vi "ProcessRepository.vi"(0 "reference in":refnum<class "Battery.lvclass">, 1 "Action(ReadRepository)":T1(ring), 5 "Error In":errorcluster) -> (7 "QueueFromProcess":refnum<queue>, 9 "ProcessViRef":refnum<vi>, 11 "ProcessSyncQueue":refnum<queue>, 13 "EventFromProcess":refnum<user-event>, 14 "reference out":refnum<class "Battery.lvclass">, 15 "EventsToProcess":refnum<user-event>, 17 "ProcessAlreadyStarted":bool, 19 "Error Out":errorcluster)   [LabVIEW 2023, in "Battery.lvclass"]
uses:
  Battery.lvclass
  Battery.lvclass/Battery.ctl
  Process.ctl
  Process.vi
panel:
  # "Use this indicator for sending messages to the Process VI"
  # "These indicators are used by the process VIs"
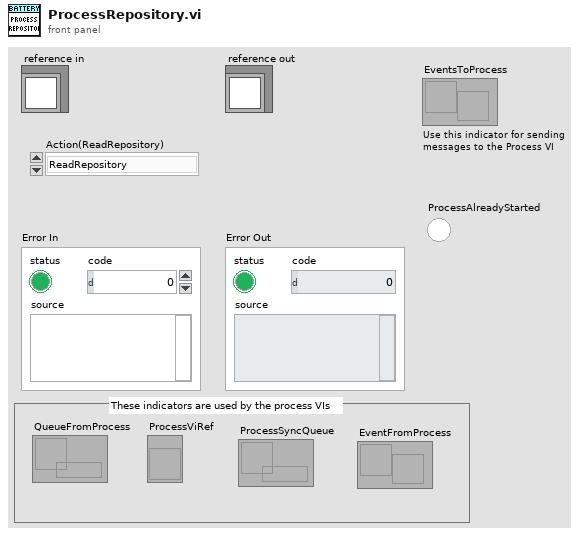
[diagram p1: front panel]
types:
  T1 = enum16{"ReadRepository", "CreateNew", "CreateOrLookUpExisting", "ReadRepositoryAndDestroy"}
  T2 = typedef "Battery.lvclass/Process.ctl" = cluster{"EventsToProcess":refnum<user-event>, "EventFromProcess":refnum<user-event>, "ProcessSyncQueue":refnum<queue>, "ProcessViRef":refnum<vi>, "QueueFromProcess":refnum<queue>}
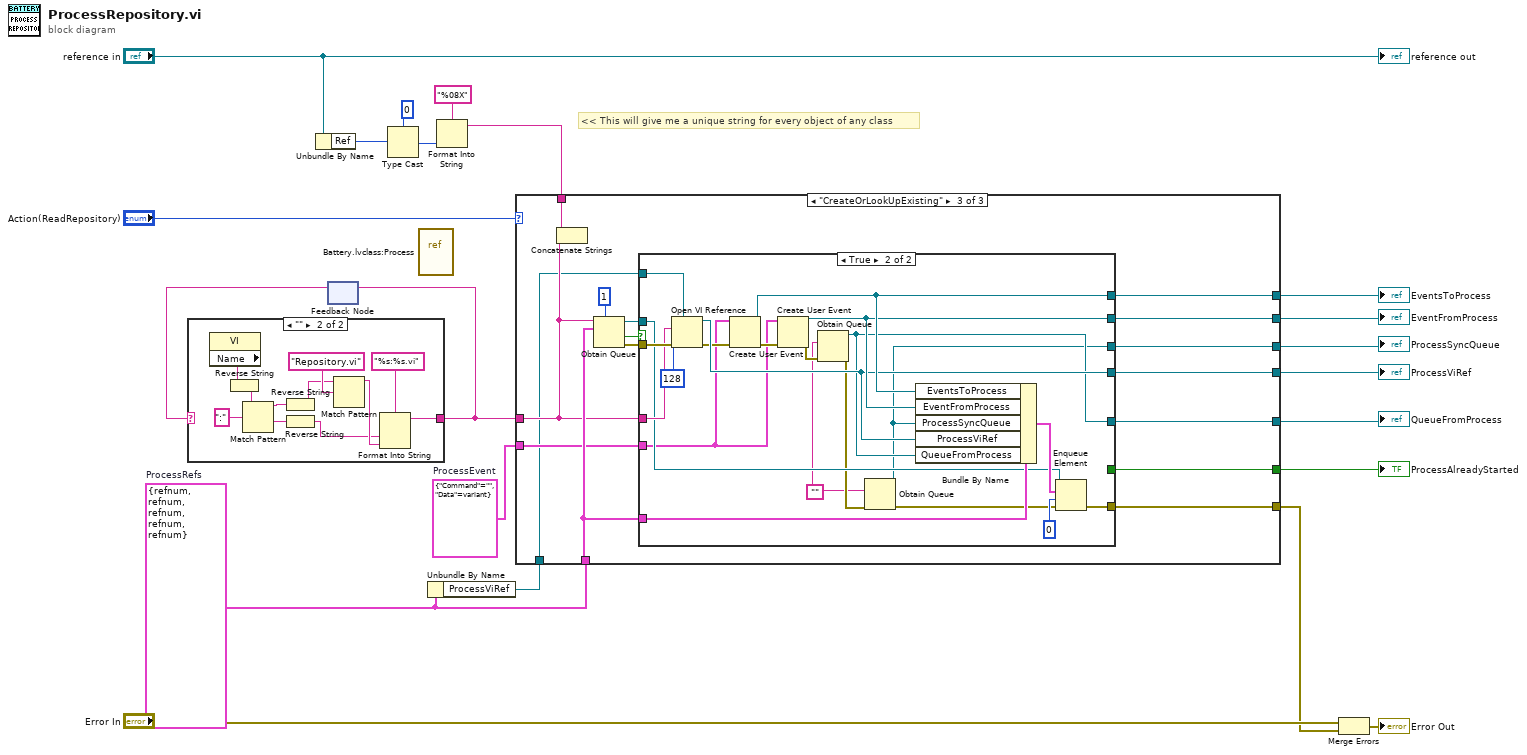
[diagram p0: block diagram]
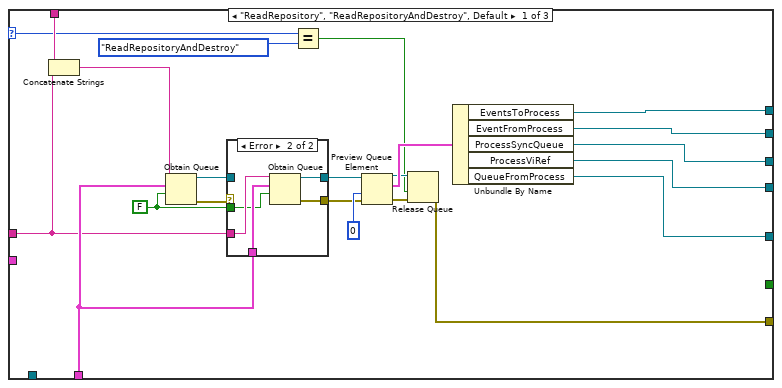
[diagram p3: hidden frame]
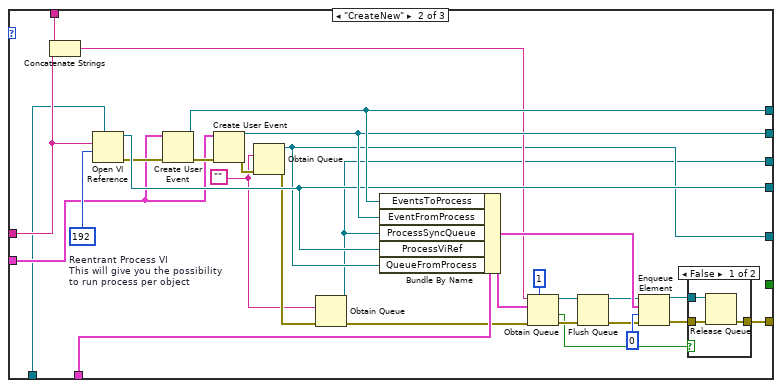
[diagram p5: hidden frame]
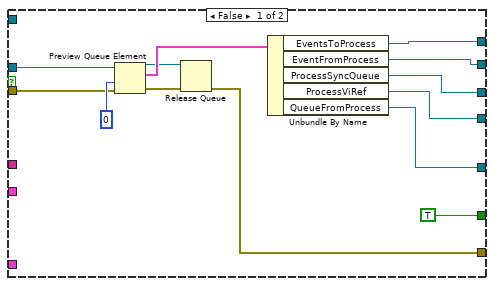
[diagram p7: hidden frame]
diagram:
  w1 = T2 {"EventsToProcess"=refnum, "EventFromProcess"=refnum, "ProcessSyncQueue"=refnum, "ProcessViRef"=refnum, "QueueFromProcess"=refnum}  # ProcessRefs
  w14 = cluster{"Command":string, "Data":variant} {"Command"="", "Data"=variant}  # ProcessEvent
  # "<< This will give me a unique string for every object of any class"
  n1 = Unbundle By Name("reference in") -> ("Ref"=w17:u32)
  n2 = feedback #1() -> (w12:string)  [unwired: 1 in]
  n3 = case shown="\"\"" w12 {
    selector: w12 -> [w22 _]
    tunnel: [w22 w23] -> w13
    frame Default {
    }
    frame "" {
      n4 = property class="VI"() -> ("Name"=w25:string)  [unwired: 2 in, 2 out]
      n5 = Reverse String(1:w25) -> (0:w26:string)
      n6 = Match Pattern(string=w26, regular expression=":") -> (before substring=w30:string, after substring=w27:string)  [unwired: 1 in, 2 out]
      n7 = Reverse String(1:w30) -> (0:w31:string)
      n8 = Reverse String(1:w27) -> (0:w29:string)
      n9 = Match Pattern(string=w31, regular expression="Repository.vi") -> (before substring=w33:string)  [unwired: 1 in, 3 out]
      n10 = Format Into String(format string="%s:%s.vi", w29, w33) -> (resulting string=w23:string)  [unwired: 2 in, 1 out]
    }
  }
  n11 = feedback-in #1(w13) -> ()
  n12 = Type Cast(type=u32 0, x=w17) -> (*(type *) &x=w20:u32)
  n13 = vi-ref "Battery.lvclass:Process.vi"() -> ()  [unwired: 1 out]
  n14 = Unbundle By Name(w1) -> ("ProcessViRef"=w11:refnum<vi>)
  n15 = Format Into String(format string="%08X", w20) -> (resulting string=w10:string)  [unwired: 2 in, 1 out]
  n16 = case shown="\"CreateOrLookUpExisting\"" "Action(ReadRepository)" {
    selector: "Action(ReadRepository)" -> [w34 _ _]
    tunnel: [w51 w71 w109] -> w5
    tunnel: [w53 w91 w111] -> w7
    tunnel: [w52 w90 w110] -> w6
    tunnel: [w54 w89 w108] -> w4
    tunnel: w1 -> [w46 w81 w104]
    tunnel: w10 -> [w44 w80 w100]
    tunnel: [w37 w64 w107] -> w8
    tunnel: w13 -> [w43 w78 w97]
    tunnel: [_ _ w102] -> w2
    tunnel: w14 -> [_ w77 w99]
    tunnel: [w41 w75 w98] -> w3
    tunnel: w11 -> [_ w63 w96]
    frame "ReadRepository", "ReadRepositoryAndDestroy", Default {
      w45 = FALSE ("create if not found? (T)")
      n17 = Concatenate Strings(w44, w43) -> (w42:string)
      n18 = Obtain Queue(name (unnamed)=w42, element data type=w46, create if not found? (T)=w45) -> (queue out=w48:refnum<queue>, error out=w50:errorcluster)  [unwired: 2 in, 1 out]
      n19 = case shown="Error" w50 {
        selector: w50 -> [w57 _]
        tunnel: [w57 w59] -> w49
        tunnel: w48 -> [w56 _]
        tunnel: [w56 w60] -> w47
        tunnel: w46 -> [_ w62]
        tunnel: w43 -> [_ w61]
        tunnel: w45 -> [_ w58]
        frame No Error {
        }
        frame Error {
          n20 = Obtain Queue(name (unnamed)=w61, element data type=w62, create if not found? (T)=w58) -> (queue out=w60:refnum<queue>, error out=w59:errorcluster)  [unwired: 2 in, 1 out]
        }
      }
      n21 = Equal?(x=w34, y=T1."ReadRepositoryAndDestroy") -> (x = y?=w35:bool)
      n22 = Preview Queue Element(queue=w47, timeout in ms (-1)=0, error in (no error)=w49) -> (queue out=w39:refnum<queue>, element=w40:T2, error out=w38:errorcluster)  [unwired: 1 out]
      n23 = Release Queue(queue=w39, force destroy? (F)=w35, error in (no error)=w38) -> (error out=w37:errorcluster)  [unwired: 2 out]
      n24 = Unbundle By Name(w40) -> ("EventsToProcess"=w53:refnum<user-event>, "EventFromProcess"=w52:refnum<user-event>, "ProcessSyncQueue"=w51:refnum<queue>, "ProcessViRef"=w54:refnum<vi>, "QueueFromProcess"=w41:refnum<queue>)
    }
    frame "CreateNew" {
      w72 = ""
      w86 = 192  # Reentrant Process VI This will give you the possibility to run process per object
      n25 = Concatenate Strings(w80, w78) -> (w79:string)
      n26 = Open VI Reference(type specifier VI Refnum (for type only)=w63, vi path=w78, options=w86) -> (vi reference=w89:refnum<vi>, error out=w87:errorcluster)  [unwired: 3 in]
      n27 = Create User Event(user event datatype=w77, error in=w87) -> (user event=w91:refnum<user-event>, error out=w88:errorcluster)
      n28 = Create User Event(user event datatype=w77, error in=w88) -> (user event=w90:refnum<user-event>, error out=w76:errorcluster)
      n29 = Obtain Queue(element data type=w72, error in (no error)=w76) -> (queue out=w75:refnum<queue>, error out=w74:errorcluster)  [unwired: 3 in, 1 out]
      n30 = Obtain Queue(element data type=w72, error in (no error)=w74) -> (queue out=w71:refnum<queue>, error out=w73:errorcluster)  [unwired: 3 in, 1 out]
      n31 = Bundle By Name(cluster=w81, "EventsToProcess"=w91, "EventFromProcess"=w90, "ProcessSyncQueue"=w71, "ProcessViRef"=w89, "QueueFromProcess"=w75) -> (w84:T2)
      n32 = Obtain Queue(max queue size (-1, unlimited)=1, name (unnamed)=w79, element data type=w84, error in (no error)=w73) -> (queue out=w85:refnum<queue>, created new?=w67:bool, error out=w69:errorcluster)  [unwired: 1 in]
      n33 = Flush Queue(queue=w85, error in (no error)=w69) -> (queue out=w70:refnum<queue>, error out=w68:errorcluster)  [unwired: 1 out]
      n34 = Enqueue Element(queue=w70, element=w84, timeout in ms (-1)=0, error in (no error)=w68) -> (queue out=w65:refnum<queue>, error out=w66:errorcluster)  [unwired: 1 out]
      n35 = case shown="False" w67 {
        tunnel: w66 -> [w94 w95]
        tunnel: w65 -> [w93 _]
        tunnel: [w92 w95] -> w64
        frame False {
          n36 = Release Queue(queue=w93, error in (no error)=w94) -> (error out=w92:errorcluster)  [unwired: 1 in, 2 out]
        }
        frame True {
        }
      }
    }
    frame "CreateOrLookUpExisting" {
      n37 = Concatenate Strings(w100, w97) -> ()  [unwired: 1 out]
      n38 = Obtain Queue(max queue size (-1, unlimited)=1, name (unnamed)=w97, element data type=w104) -> (queue out=w105:refnum<queue>, created new?=w106:bool, error out=w103:errorcluster)  [unwired: 2 in]
      n39 = case shown="True" w106 {
        tunnel: [w124 w145] -> w111
        tunnel: [w123 w144] -> w110
        tunnel: [w122 w128] -> w109
        tunnel: [w121 w143] -> w108
        tunnel: [w112 w142] -> w107
        tunnel: w104 -> [_ w141]
        tunnel: w103 -> [w118 w136]
        tunnel: w97 -> [_ w135]
        tunnel: w105 -> [w119 w134]
        tunnel: [TRUE _] -> w102
        tunnel: w99 -> [_ w133]
        tunnel: [w115 w131] -> w98
        tunnel: w96 -> [_ w126]
        frame False {
          n40 = Preview Queue Element(queue=w119, timeout in ms (-1)=0, error in (no error)=w118) -> (queue out=w114:refnum<queue>, element=w117:T2, error out=w113:errorcluster)  [unwired: 1 out]
          n41 = Release Queue(queue=w114, error in (no error)=w113) -> (error out=w112:errorcluster)  [unwired: 1 in, 2 out]
          n42 = Unbundle By Name(w117) -> ("EventsToProcess"=w124:refnum<user-event>, "EventFromProcess"=w123:refnum<user-event>, "ProcessSyncQueue"=w122:refnum<queue>, "ProcessViRef"=w121:refnum<vi>, "QueueFromProcess"=w115:refnum<queue>)
        }
        frame True {
          w129 = ""
          n43 = Open VI Reference(type specifier VI Refnum (for type only)=w126, vi path=w135, options=128, error in (no error)=w136) -> (vi reference=w143:refnum<vi>, error out=w139:errorcluster)  [unwired: 2 in]
          n44 = Create User Event(user event datatype=w133, error in=w139) -> (user event=w145:refnum<user-event>, error out=w140:errorcluster)
          n45 = Create User Event(user event datatype=w133, error in=w140) -> (user event=w144:refnum<user-event>, error out=w132:errorcluster)
          n46 = Obtain Queue(element data type=w129, error in (no error)=w132) -> (queue out=w131:refnum<queue>, error out=w130:errorcluster)  [unwired: 3 in, 1 out]
          n47 = Obtain Queue(element data type=w129, error in (no error)=w130) -> (queue out=w128:refnum<queue>, error out=w127:errorcluster)  [unwired: 3 in, 1 out]
          n48 = Bundle By Name(cluster=w141, "EventsToProcess"=w145, "EventFromProcess"=w144, "ProcessSyncQueue"=w128, "ProcessViRef"=w143, "QueueFromProcess"=w131) -> (w138:T2)
          n49 = Enqueue Element(queue=w134, element=w138, timeout in ms (-1)=0, error in (no error)=w127) -> (error out=w142:errorcluster)  [unwired: 2 out]
        }
      }
    }
  }
  "ProcessSyncQueue" <- w5
  "EventsToProcess" <- w7
  "EventFromProcess" <- w6
  "ProcessViRef" <- w4
  "ProcessAlreadyStarted" <- w2
  "QueueFromProcess" <- w3
  n50 = Merge Errors("Error In", w8) -> (→"Error Out":errorcluster)
  "reference out" <- "reference in"
